vi "AFO_NLF.vi"() -> ()   [LabVIEW 2016]
uses:
  <vilib>/myRIO/Common/Instrument Driver Framework/myRIO v1.0/Encoder/typedefs/Encoder Signal Mode.ctl
  <vilib>/Platform/TimedLoop/XDataNode/timing_clust.ctl
  <vilib>/Platform/TimedLoop/XDataNode/nitl_modes.ctl
  <vilib>/Platform/TimedLoop/XDataNode/wakeup.ctl
  <vilib>/myRIO/Common/Instrument Driver Framework/myRIO v1.0/UART/vis/myRIO v1.0 Close UART.vi
  <vilib>/Utility/file.llb/Write Delimited Spreadsheet (DBL).vi
  <vilib>/Utility/error.llb/Error Cluster From Error Code.vi
  <vilib>/myRIO/Common/Instrument Driver Framework/myRIO v1.0/Encoder/vis/myRIO v1.0 Read Encoder.vi
  <vilib>/imath/engines/lvmath2/RunTimeEngine/ArithmeticOperatorToken/NIMS_ArithmeticOperator_times.vi
  <instcachedir>/0/NIMS_ArithmeticOperator_times_953B34F74CAC448FB707D816A29CC5F0.lvgen/NIMS_ArithmeticOperator_times_953B34F74CAC448FB707D816A29CC5F0_000.vi
  <vilib>/imath/engines/lvmath2/RunTimeEngine/BuiltInFunctions/sum/NIMS_sum(GV).vi
  <instcachedir>/0/NIMS_sum(GV)_67F5EC36BC034E54A6BEC5B0673C00E5.lvgen/NIMS_sum(GV)_67F5EC36BC034E54A6BEC5B0673C00E5_000.vi
  <vilib>/imathl/engines/lvmath/Functions/Error Handling/Create Error.vi
  <vilib>/imath/engines/lvmath2/RunTimeEngine/RangeToken/NIMS_Range.vi
  <instcachedir>/0/NIMS_Range_A7C094595B484CA7AF10685B02D808ED.lvgen/NIMS_Range_A7C094595B484CA7AF10685B02D808ED_001.vi
  <instcachedir>/0/NIMS_ArithmeticOperator_times_953B34F74CAC448FB707D816A29CC5F0.lvgen/NIMS_ArithmeticOperator_times_953B34F74CAC448FB707D816A29CC5F0_008.vi
  <vilib>/imath/engines/lvmath2/RunTimeEngine/ArithmeticOperatorToken/NIMS_ArithmeticOperator_plus.vi
  <instcachedir>/0/NIMS_ArithmeticOperator_plus_0120E0498A0F4B4B9BDCAC2554767A4E.lvgen/NIMS_ArithmeticOperator_plus_0120E0498A0F4B4B9BDCAC2554767A4E_004.vi
  <vilib>/imath/engines/lvmath2/RunTimeEngine/ErrorHandling/NIMS_Create Error From Enums.vi
  <vilib>/imath/engines/lvmath2/RunTimeEngine/BuiltInFunctions/mod/NIMS_mod_no_size_check.vi
  <instcachedir>/0/NIMS_mod_no_size_check_5393E3382FD241D281EEB71DA286C65B.lvgen/NIMS_mod_no_size_check_5393E3382FD241D281EEB71DA286C65B_008.vi
  <vilib>/imath/engines/lvmath2/RunTimeEngine/IndexRead/NIMS V(S).vi
  <instcachedir>/0/NIMS V(S)_0488751826AF41519A22953C041130DC.lvgen/NIMS V(S)_0488751826AF41519A22953C041130DC_000.vi
  <vilib>/imath/engines/lvmath2/RunTimeEngine/ArithmeticOperatorToken/NIMS_ArithmeticOperator_minus.vi
  <instcachedir>/0/NIMS_ArithmeticOperator_minus_E3B65B1D26A44BB184AFDC5B3F458E3D.lvgen/NIMS_ArithmeticOperator_minus_E3B65B1D26A44BB184AFDC5B3F458E3D_003.vi
  <vilib>/imath/engines/lvmath/Functions/Error Handling/MergeErrorsWrapper.vi
  <vilib>/imath/engines/lvmath2/RunTimeEngine/ArithmeticOperatorToken/NIMS_ArithmeticOperator_rightdiv.vi
  <instcachedir>/0/NIMS_ArithmeticOperator_rightdiv_0403F5D95ED04A4080FE3DA43A6A83B7.lvgen/NIMS_ArithmeticOperator_rightdiv_0403F5D95ED04A4080FE3DA43A6A83B7_000.vi
  <vilib>/imath/engines/lvmath2/RunTimeEngine/NodeEndStatement/NIMS_NodeEndStatement_Output.vi
  <instcachedir>/0/NIMS_NodeEndStatement_Output_53EC0D466D134D7ABD903AC30B43404B.lvgen/NIMS_NodeEndStatement_Output_53EC0D466D134D7ABD903AC30B43404B_005.vi
  <instcachedir>/0/NIMS_NodeEndStatement_Output_53EC0D466D134D7ABD903AC30B43404B.lvgen/NIMS_NodeEndStatement_Output_53EC0D466D134D7ABD903AC30B43404B_001.vi
  <vilib>/imath/engines/lvmath2/RunTimeEngine/ErrorHandling/NIMS_Finalize Error.vi
  <vilib>/myRIO/Common/Instrument Driver Framework/Utilities/vis/FPGA Ref Manager.vi
  <vilib>/myRIO/Common/Instrument Driver Framework/myRIO v1.0/myRIO v1.0 Reset FPGA.vi
  <vilib>/myRIO/Common/Instrument Driver Framework/myRIO v1.0/IRQ/vis/myRIO v1.0 IRQ Info FGV.vi
  <vilib>/myRIO/Common/Instrument Driver Framework/myRIO v1.0/IRQ/vis/myRIO v1.0 Timer IRQ Info FGV.vi
  <vilib>/myRIO/Common/Instrument Driver Framework/myRIO v1.0/IRQ/vis/myRIO v1.0 ISR Agent.vi
  <vilib>/platform/TimedLoop/XDataNode/XDataNode.xnode
  <vilib>/myRIO/Instrument Drivers/Onboard IO/Encoder/Encoder.lvlib
  <vilib>/myRIO/Instrument Drivers/Utilities/Utilities.lvlib
  <vilib>/Platform/TimedLoop/XDataNode/XDNodeRunTimeDep.lvlib
panel:
  out "Counter Value 3":dbl(graph)
  out "Finished Late? [i-1]":bool
  out "Counter Value 2":T1(graph)
  in  "stop 2":bool
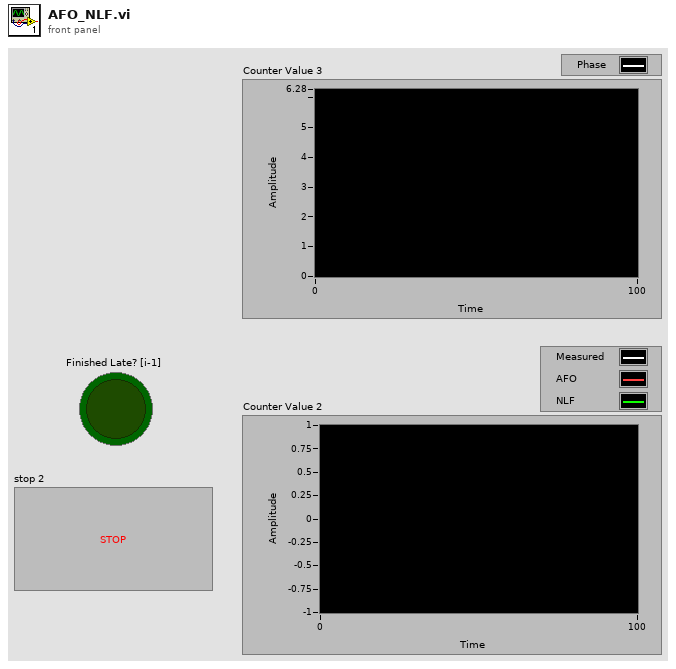
[diagram p1: front panel]
types:
  T1 = cluster{"q_RA":dbl, "theta_hat":dbl, "theta_tilde":dbl}
  T2 = typedef "XDNodeRunTimeDep.lvlib/timing_clust.ctl" = cluster{"Expected End [f-1]":u64, "Actual End [f-1]":u64, "Finished Late? [f-1]":bool, "Expected End [i-1]":u64, "Actual End [i-1]":u64, "Finished Late? [i-1]":bool, "Expected Start [i]":u64, "Actual Start [i]":u64, "Expected Start [f]":u64, "Actual Start [f]":u64, "Source Name":string, "Structure Name":string, "Period":i64, "Deadline":i64, "Offset":i64, "Start":i64, "Priority":i32, "Timeout":i32, "Mode":T3, "Wakeup Reason":T4, "Error":errorcluster, "Source Type":string, "Secondary Source Type":string, "Global End Time":u64, "Global Start Time":u64, "Frame Duration":u64, "Iteration Duration":u64, "Assigned CPU":i32, "I/O Scan Engine Mode":u32}
  T3 = typedef "XDNodeRunTimeDep.lvlib/nitl_modes.ctl" = enum32{"No Change", "Process missed periods, maintain original phase", "Discard missed periods, maintain original phase", "Process missed periods, ignore original phase", "Discard missed periods, ignore original phase"}
  T4 = typedef "XDNodeRunTimeDep.lvlib/wakeup.ctl" = enum32{"Normal", "Aborted", "Asynchronous wakeup", "Timing source error", "Timed loop error", "Timeout"}
  T5 = typedef "Encoder Signal Mode.ctl" = enum16{"Quadrature phase signal", "Step and direction signal"}
  T6 = typedef "Encoder.lvlib/Encoder Reference.ctl" = cluster{"myRIO Reference":T7, "Encoder Channels Enum":T11}
  T7 = typedef "myRIO Generic Hardware Reference.ctl" = cluster{"myRIO Model":T8, "myRIO Hardware Reference":T9}
  T8 = typedef "Hardware Version Enum.ctl" = enum16{"Unknown", "myRIO-1900", "myRIO-1950", "roboRIO", "NI ELVIS RIO CM"}
  T9 = typedef "myRIO v1.0 Reference.ctl" = cluster{"Generic FPGA Reference":T10, "Allow multiple opens":bool}
  T10 = typedef "Generic FPGA Reference.ctl" = refnum<k20>
  T11 = typedef "Encoder Channels Enum.ctl" = enum16{"Not Connected", "C/ENC0", "C/ENC1", "A/ENC", "B/ENC", "DIO/ENC0", "DIO/ENC1", "DIO/ENC2", "DIO/ENC3", "DIO/ENC4"}
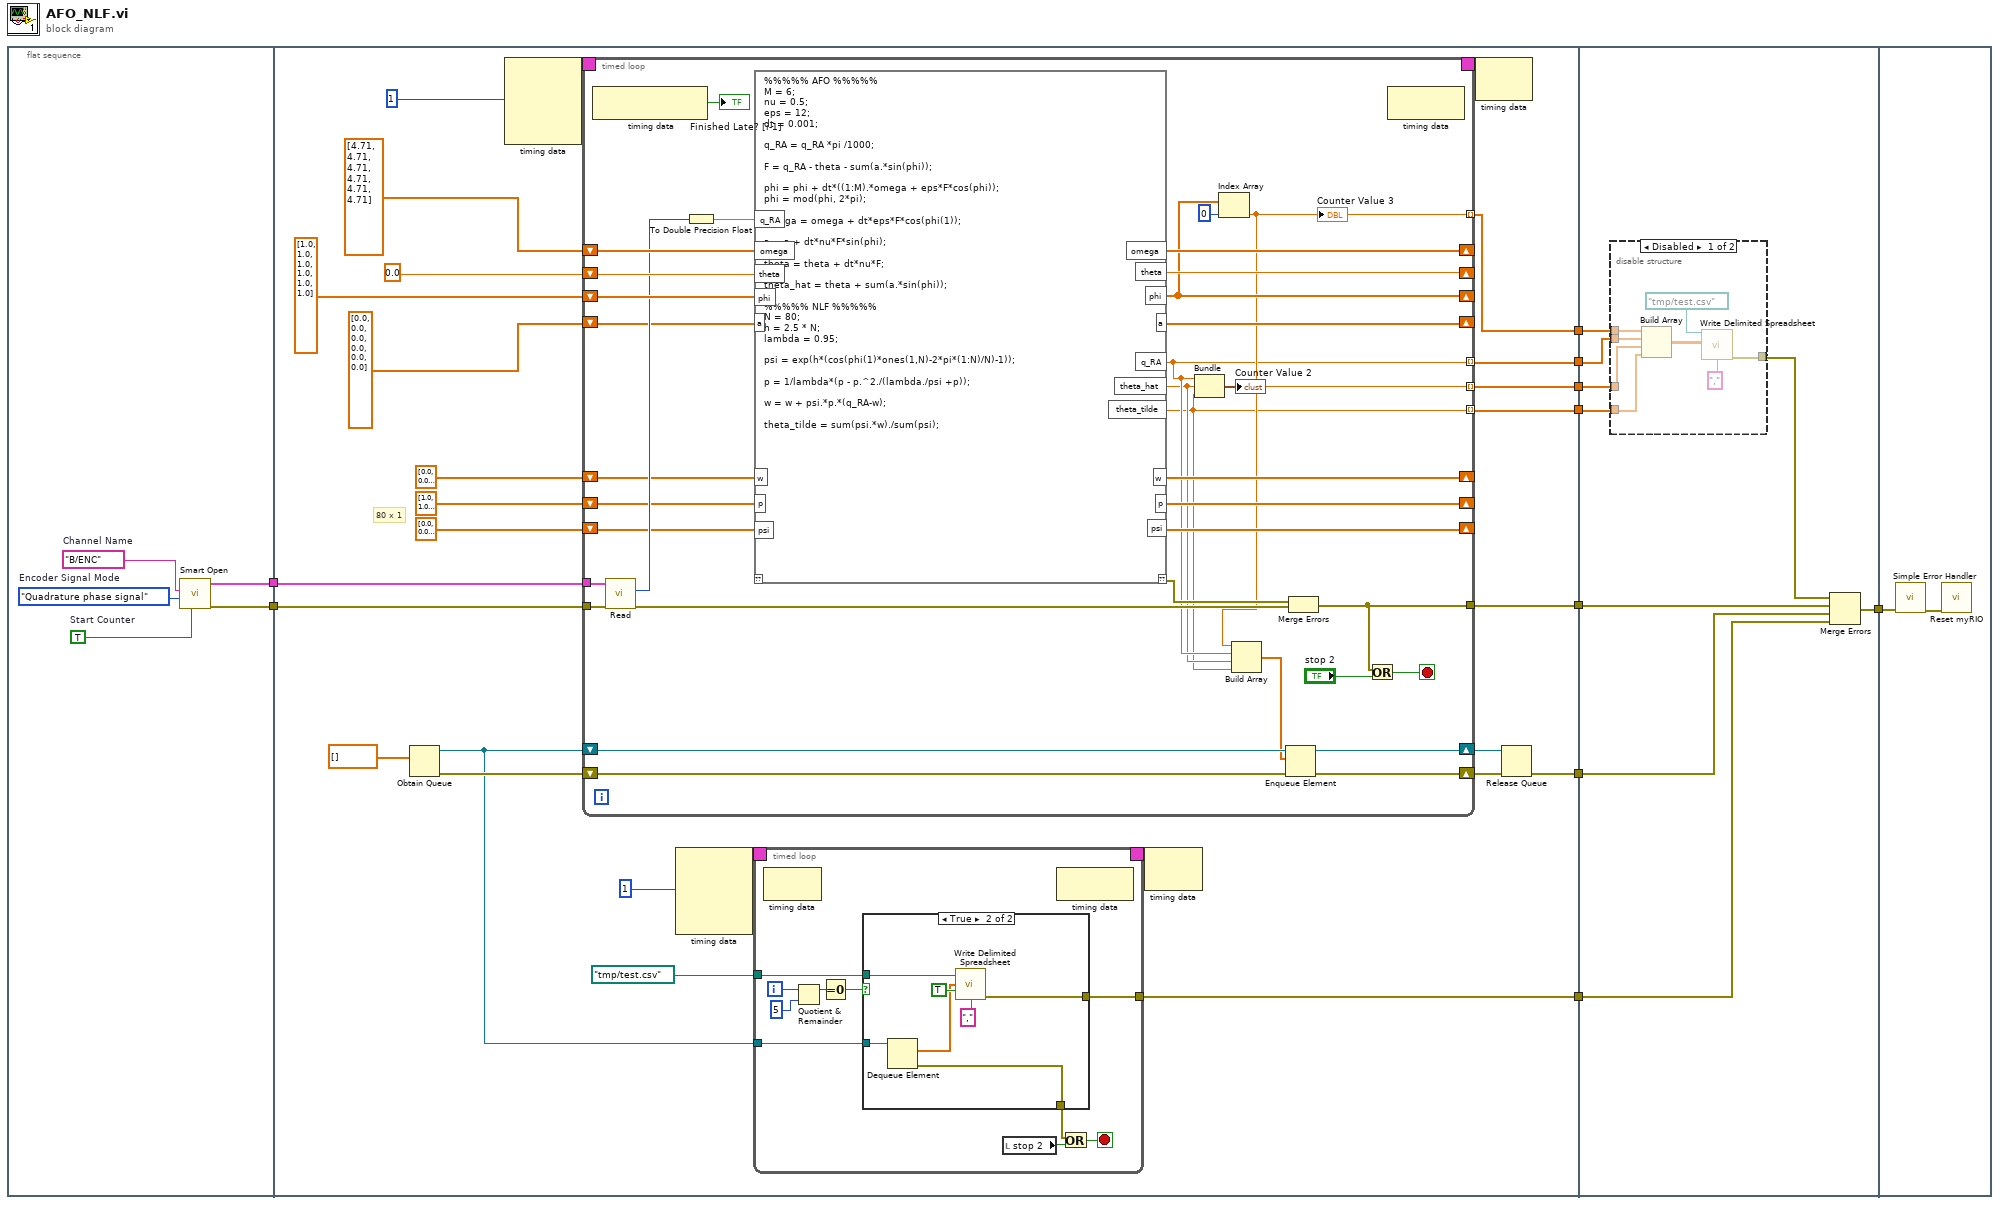
[diagram p0: block diagram]
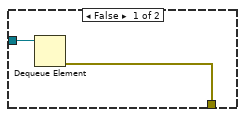
[diagram p2: hidden frame]
diagram:
  n1 = flat-sequence {
    tunnel: [w12] -> w10
    tunnel: [w11] -> w9
    tunnel: w10 -> [w43]
    tunnel: w9 -> [w42]
    tunnel: [w41] -> w8
    tunnel: [w30] -> w6
    tunnel: [w29] -> w5
    tunnel: [w28] -> w4
    tunnel: [w27] -> w3
    tunnel: [w22] -> w2
    tunnel: [w16] -> w1
    tunnel: [w503] -> w7
    tunnel: w8 -> [w502]
    tunnel: w6 -> [w501]
    tunnel: w5 -> [w500]
    tunnel: w4 -> [w499]
    tunnel: w3 -> [w498]
    tunnel: w2 -> [w497]
    tunnel: w1 -> [w496]
    tunnel: w7 -> [w512]
    frame #0 {
      w13 = TRUE  # Start Counter
      w14 = Encoder_Signal_Mode."Quadrature phase signal"  # Encoder Signal Mode
      w15 = tag "B/ENC"  # Channel Name
      n2 = call <vilib>:"Smart Open.vi"("Start Counter"=w13, "Encoder Signal Mode"=w14, "Channel Name"=w15) -> ("error out"=w11:errorcluster, "Encoder Ref Out"=w12:T6)  [unwired: 7 in]
    }
    frame #1 {
      # "80 x 1"
      n3 = Obtain Queue(element data type=dbl[] []) -> (queue out=w21:refnum<queue>, error out=w24:errorcluster)  [unwired: 4 in, 1 out]
      n4 = node-c288(i64 1 ("Period")) -> (w40:T2)  [unwired: 3 in]
      n5 = timed-loop {
        tunnel: w43 -> [w103]
        tunnel: w42 -> [w102]
        tunnel: [w96] -> w41
        timing: w40 -> [_]
        timing-out: [_] -> w39
        shift-right: [w89] -> _
        shift-left: dbl[] [4.71, 4.71, 4.71, 4.71, 4.71, 4.71] -> [w94]
        shift-right: [w90] -> _
        shift-left: 0.0 ("omega") -> [w93]
        shift-right: [w88] -> _
        shift-left: dbl[] [1.0, 1.0, 1.0, 1.0, 1.0, 1.0] -> [w92]
        shift-right: [w91] -> _
        shift-left: dbl[] [0.0, 0.0, 0.0, 0.0, 0.0, 0.0] -> [w78]
        shift-right: [w82] -> _
        shift-left: dbl[] [0.0, 0.0, 0.0, 0.0, 0.0, 0.0, 0.0, 0.0, 0.0, 0.0, 0.0, 0.0, 0.0, 0.0, 0.0, 0.0, 0.0, 0.0, 0.0, 0.0, 0.0, 0.0, 0.0, 0.0, 0.0, 0.0, 0.0, 0.0, 0.0, 0.0, 0.0, 0.0, 0.0, 0.0, 0.0, 0.0, 0.0, 0.0, 0.0, 0.0, 0.0, 0.0, 0.0, 0.0, 0.0, 0.0, 0.0, 0.0, 0.0, 0.0, 0.0, 0.0, 0.0, 0.0, 0.0, 0.0, 0.0, 0.0, 0.0, 0.0, 0.0, 0.0, 0.0, 0.0, 0.0, 0.0, 0.0, 0.0, 0.0, 0.0, 0.0, 0.0, 0.0, 0.0, 0.0, 0.0, 0.0, 0.0, 0.0, 0.0] -> [w84]
        shift-right: [w80] -> _
        shift-left: dbl[] [0.0, 0.0, 0.0, 0.0, 0.0, 0.0, 0.0, 0.0, 0.0, 0.0, 0.0, 0.0, 0.0, 0.0, 0.0, 0.0, 0.0, 0.0, 0.0, 0.0, 0.0, 0.0, 0.0, 0.0, 0.0, 0.0, 0.0, 0.0, 0.0, 0.0, 0.0, 0.0, 0.0, 0.0, 0.0, 0.0, 0.0, 0.0, 0.0, 0.0, 0.0, 0.0, 0.0, 0.0, 0.0, 0.0, 0.0, 0.0, 0.0, 0.0, 0.0, 0.0, 0.0, 0.0, 0.0, 0.0, 0.0, 0.0, 0.0, 0.0, 0.0, 0.0, 0.0, 0.0, 0.0, 0.0, 0.0, 0.0, 0.0, 0.0, 0.0, 0.0, 0.0, 0.0, 0.0, 0.0, 0.0, 0.0, 0.0, 0.0] -> [w79]
        shift-right: [w81] -> _
        shift-left: dbl[] [1.0, 1.0, 1.0, 1.0, 1.0, 1.0, 1.0, 1.0, 1.0, 1.0, 1.0, 1.0, 1.0, 1.0, 1.0, 1.0, 1.0, 1.0, 1.0, 1.0, 1.0, 1.0, 1.0, 1.0, 1.0, 1.0, 1.0, 1.0, 1.0, 1.0, 1.0, 1.0, 1.0, 1.0, 1.0, 1.0, 1.0, 1.0, 1.0, 1.0, 1.0, 1.0, 1.0, 1.0, 1.0, 1.0, 1.0, 1.0, 1.0, 1.0, 1.0, 1.0, 1.0, 1.0, 1.0, 1.0, 1.0, 1.0, 1.0, 1.0, 1.0, 1.0, 1.0, 1.0, 1.0, 1.0, 1.0, 1.0, 1.0, 1.0, 1.0, 1.0, 1.0, 1.0, 1.0, 1.0, 1.0, 1.0, 1.0, 1.0] -> [w83]
        tunnel: [w72] -> w27 mode=indexing
        tunnel: [w73] -> w28 mode=indexing
        tunnel: [w74] -> w29 mode=indexing
        tunnel: [w75] -> w30 mode=indexing
        shift-right: [w76] -> w26
        shift-left: w21 -> [w77]
        shift-right: [w69] -> w23
        shift-left: w24 -> [w70]
        stop <- w95 stop-if-true
        n6 = node-c288() -> (→"Finished Late? [i-1]":bool)  [unwired: 1 in]
        n7 = call <vilib>:"Read.vi"("error in (no error)"=w102, "Encoder Ref In"=w103) -> ("error out"=w98:errorcluster, "Counter Value"=w85:i32)  [unwired: 5 in, 3 out]
        n8 = To Double Precision Float(number=w85) -> (double precision float=w100:dbl)
        n9 = mathscript code="%%%%% AFO %%%%%\nM = 6;\nnu = 0.5;\neps = 12;\ndt = 0.001;\n\nq_RA = q_RA *pi /1000;\n\nF = q_RA - theta - sum(a.*sin(phi));\n\nphi = phi + dt*((1:M).*omega + eps*F*cos(phi));\nphi = mod(phi, 2*pi);\n\nomega = omega + dt*eps*F*cos(phi(1));\n\na = a + dt*nu*F*sin(phi);\n\ntheta = theta + dt*nu*F;\n\ntheta_hat = theta + sum(a.*sin(phi));\n\n%%%%% NLF %%%%%\nN = 80;\nh = 2.5 * N;\nlambda = 0.95;\n\npsi = exp(h*(cos(phi(1)*ones(1,N)-2*pi*(1:N)/N)-1));\n\np = 1/lambda*(p - p.^2./(lambda./psi +p));\n\nw = w + psi.*p.*(q_RA-w);\n\ntheta_tilde = sum(psi.*w)./sum(psi);"("q_RA"=w100, "omega"=w94, "theta"=w93, "phi"=w92, "a"=w78, "w"=w84, "p"=w83, "psi"=w79) -> ("??"=w99:errorcluster, "omega"=w89:dbl[], "theta"=w90:dbl, "a"=w91:dbl[], "phi"=w88:dbl[], "theta_hat"=w73:dbl, "q_RA"=w74:dbl, "theta_tilde"=w72:dbl, "w"=w82:dbl[], "p"=w81:dbl[], "psi"=w80:dbl[])  [unwired: 1 in]
        n10 = Bundle("q_RA"=w74, "theta_hat"=w73, "theta_tilde"=w72) -> (→"Counter Value 2":T1)  [unwired: 1 in]
        n11 = Index Array(array=w88, index=0) -> (element=w75:dbl)
        "Counter Value 3" <- w75
        n12 = Build Array(w75, w74, w73, w72) -> (w71:dbl[])
        n13 = Enqueue Element(queue=w77, element=w71, error in (no error)=w70) -> (queue out=w76:refnum<queue>, error out=w69:errorcluster)  [unwired: 1 in, 1 out]
        n14 = Merge Errors(w99, w98) -> (w96:errorcluster)
        n15 = Or(x=w96, y="stop 2") -> (x .or. y?=w95:bool)
        n16 = node-c288() -> ()  [unwired: 1 in, 1 out]
      }
      n17 = node-c288(i64 1 ("Period")) -> (w20:T2)  [unwired: 3 in]
      n18 = timed-loop {
        tunnel: w21 -> [w51]
        timing: w20 -> [_]
        timing-out: [_] -> w19
        tunnel: path "/tmp/test.csv" ("file path (dialog if empty)") -> [w45]
        tunnel: [w44] -> w16
        i -> [w49]
        stop <- w52 stop-if-true
        n19 = node-c288() -> ()  [unwired: 1 in, 1 out]
        n20 = Quotient & Remainder(x=w49, y=5) -> (x-y*floor(x/y)=w47:i32)  [unwired: 1 out]
        n21 = Equal To 0?(x=w47) -> (x = 0?=w46:bool)
        n22 = case shown="True" w46 {
          tunnel: w51 -> [w55 w62]
          tunnel: [w54 w61] -> w50
          tunnel: w45 -> [_ w60]
          tunnel: [_ w56] -> w44
          frame False {
            n23 = Dequeue Element(queue=w55) -> (error out=w54:errorcluster)  [unwired: 2 in, 3 out]
          }
          frame True {
            n24 = Dequeue Element(queue=w62) -> (element=w57:dbl[], error out=w61:errorcluster)  [unwired: 2 in, 2 out]
            n25 = call-poly <vilib>:"Write Delimited Spreadsheet.vi"("file path (dialog if empty)"=w60, "1D data"=w57, "append to file? (new file:F)"=TRUE, "delimiter (\\t)"="," ("delimiter (\\t)")) -> ("error out"=w56:errorcluster)  [unwired: 10 in, 1 out]
          }
        }
        n26 = local read "stop 2"() -> (w53:bool)
        n27 = node-c288() -> ()  [unwired: 1 in, 1 out]
        n28 = Or(x=w50, y=w53) -> (x .or. y?=w52:bool)
      }
      n29 = node-c288(w19) -> ()  [unwired: 1 out]
      n30 = node-c288(w39) -> ()  [unwired: 1 out]
      n31 = Release Queue(queue=w26, error in (no error)=w23) -> (error out=w22:errorcluster)  [unwired: 1 in, 2 out]
    }
    frame #2 {
      n32 = disable-structure shown="Disabled" {
        disable-tunnel: w501 -> [w511 _]
        disable-tunnel: w500 -> [w510 _]
        disable-tunnel: w499 -> [w509 _]
        disable-tunnel: w498 -> [w508 _]
        disable-tunnel: [w505 _] -> w495
        frame Disabled {
          n33 = Build Array(w511, w510, w509, w508) -> (w507:dbl[][])
          n34 = call-poly <vilib>:"Write Delimited Spreadsheet.vi"("file path (dialog if empty)"=path "/tmp/test.csv", "2D data"=w507, "delimiter (\\t)"="," ("delimiter (\\t)")) -> ("error out"=w505:errorcluster)  [unwired: 11 in, 1 out]
        }
        frame Enabled {
        }
      }
      n35 = Merge Errors(w495, w502, w497, w496) -> (w503:errorcluster)
    }
    frame #3 {
      n36 = call <vilib>:"Simple Error Handler.vi"("error in (no error)"=w512) -> ("error out"=w513:errorcluster)  [unwired: 4 in, 4 out]
      n37 = call <vilib>:"Reset myRIO.vi"("error in (no error)"=w513) -> ()  [unwired: 10 in, 1 out]
    }
  }
